vi "Create new save file.vi"(2 "Insert":string, 3 "Ext":string=".dat", 4 "Index In":dbl=1.0) -> (0 "Path Out":path, 1 "Index Out":dbl)   [LabVIEW 2014]
panel:
  in  "Folder":string="P:\\Data\\"
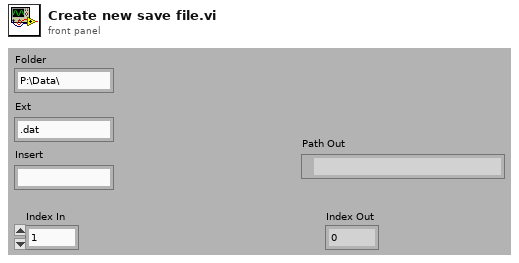
[diagram p1: front panel]
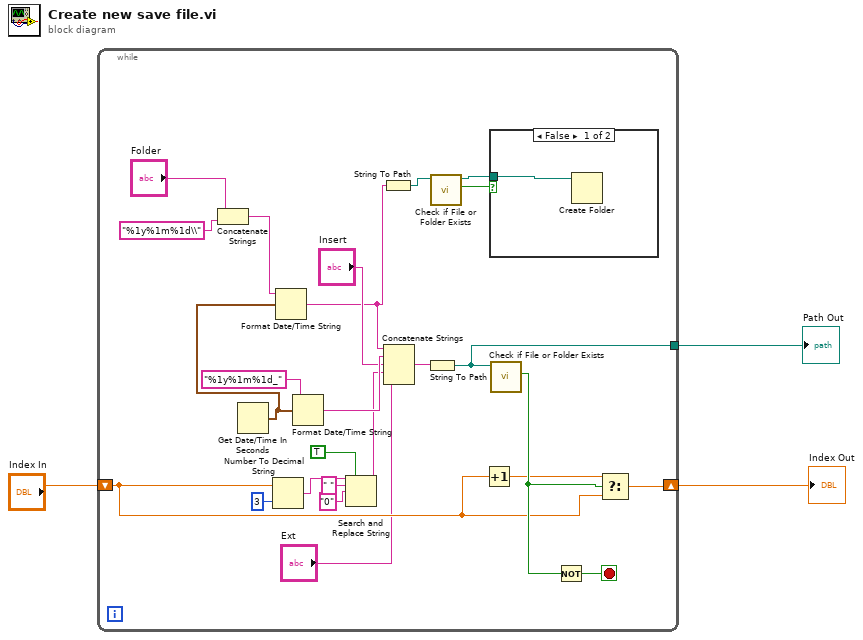
[diagram p0: block diagram]
diagram:
  n1 = while {
    tunnel: [w22] -> w2
    shift-right: [w20] -> w1
    shift-left: "Index In" -> [w18]
    stop <- w21 stop-if-true
    n2 = Concatenate Strings("Folder", "%1y%1m%1d\\" ("time format string (%c)")) -> (w4:string)
    n3 = Get Date/Time In Seconds() -> (seconds since 1Jan1904=w14:timestamp)
    n4 = Number To Decimal String(number=w18, width (-)=i16 3) -> (decimal integer string=w24:string)
    n5 = Format Date/Time String(time format string (%c)=w4, seconds (now)=w14) -> (date/time string=w10:string)  [unwired: 1 out]
    n6 = Format Date/Time String(time format string (%c)="%1y%1m%1d_", seconds (now)=w14) -> (date/time string=w27:string)  [unwired: 1 out]
    n7 = Search and Replace String(replace all?=TRUE ("replace all? (F)"), input string=w24, search string=" ", replace string="0" ("replace string (\"\")")) -> (result string=w13:string)  [unwired: 1 in, 6 out]
    n8 = String To Path(string=w10) -> (path=w9:path)
    n9 = Concatenate Strings(w10, w27, "Insert", w13, "Ext") -> (w28:string)
    n10 = String To Path(string=w28) -> (path=w22:path)
    n11 = call <vilib>:"Check if File or Folder Exists.vi"("path"=w9) -> ("file or folder exists?"=w8:bool, "dup path"=w7:path)  [unwired: 1 in, 8 out]
    n12 = Increment(x=w18) -> (x+1=w17:dbl)
    n13 = case shown="False" w8 {
      tunnel: w7 -> [w29 _]
      frame False {
        n14 = Create Folder(path (use dialog)=w29) -> ()  [unwired: 1 in, 4 out]
      }
      frame True {
      }
    }
    n15 = call <vilib>:"Check if File or Folder Exists.vi"("path"=w22) -> ("file or folder exists?"=w19:bool)  [unwired: 1 in, 9 out]
    n16 = Not(x=w19) -> (.not. x?=w21:bool)
    n17 = Select(t=w17, s=w19, f=w18) -> (s? t:f=w20:dbl)
  }
  "Index Out" <- w1
  "Path Out" <- w2
